vi "run method.vi"(8 "error in (no error)":errorcluster, 10 "VI in":refnum<vi>, 11 "JSON Value in":refnum<class "JSON Value.lvclass">) -> (0 "error out":errorcluster, 3 "JSON Value out":refnum<class "JSON Value.lvclass">)   [LabVIEW 2017]
uses:
  <vilib>/NI/JSON Support for LabVIEW/JSON Value/JSON Value.lvclass
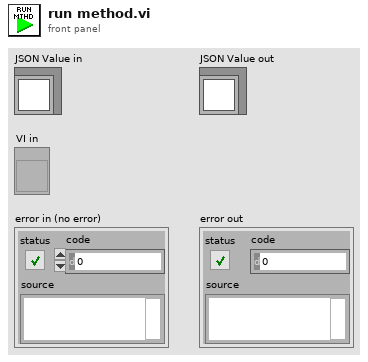
[diagram p1: front panel]
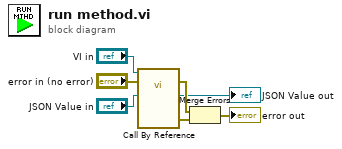
[diagram p0: block diagram]
diagram:
  n1 = call-by-ref "?"(reference="VI in", error in="error in (no error)", "params"="JSON Value in") -> (error out=w4:errorcluster, 0:"error out"=w5:errorcluster, "data"=→"JSON Value out":refnum<class "JSON Value.lvclass">)  [unwired: 9 in, 1 out]
  n2 = Merge Errors(w4, w5) -> (→"error out":errorcluster)
